vi "Dlg-Add-Exchanges.vi"(8 "error in (no error)":errorcluster, 11 "Exchanges in":refnum<class "Exchanges.lvclass">) -> (0 "error out":errorcluster, 2 "Canceled":bool, 3 "Exchanges out":refnum<class "Exchanges.lvclass">)   [LabVIEW 2012]
uses:
  Exchange/Exchange.lvclass
  Exchange/Exchange Type Enum.ctl
  controls/Currencies.ctl
  Exchange/Exchange Parameters.ctl
  Exchanges.lvclass
  Stocks Manager/Stock Manager Action.ctl
panel:
  in  "Label":string
  in  "ISIN":string
  in  "Taxe":dbl
  in  "Quantité":dbl
  in  "Type":T1
  in  "Currency":T2
  in  "Prix":dbl
  in  "Add":bool
  in  "Date":timestamp format="%<%X\n%x>T"
  in  "Commentaires":string
  in  "Cancel Button":bool
  in  "Help":bool
  # "Nouveau Portefeuille"
  # "Ajouter une Transaction"
  # "Transaction"
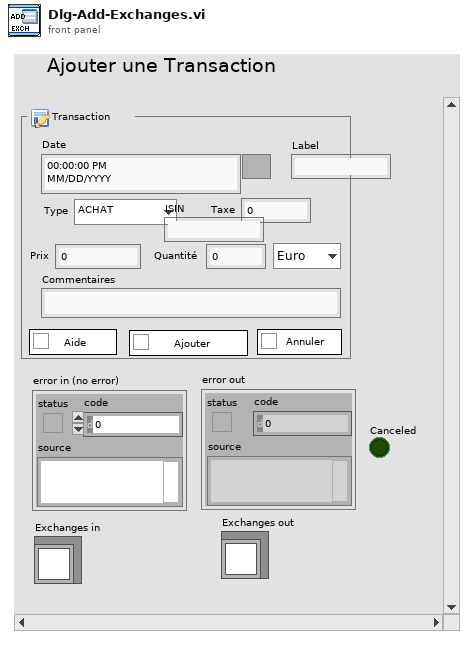
[diagram p1: front panel]
types:
  T1 = typedef "Exchange.lvclass/Exchange Type Enum.ctl" = enum16{"ACHAT", "VENTE"}
  T2 = typedef "Currencies.ctl" = enum16{"Euro", "Dollar", "Yen", "RIM", "CHF"}
  T3 = typedef "Exchange Parameters.ctl" = cluster{"Date":timestamp, "Exchange Type":T1, "ISIN":string, "Label":string, "Price":dbl, "Qty":dbl, "Currency":T2, "Tax":dbl, "Comment":string}
  T4 = typedef "Stock Manager Action.ctl" = enum16{"Get_Stocks", "Load_Stocks", "Find_Stock_From_ISIN", "Find_Stock_From_Label", "Find_Stock_From_Symbol"}
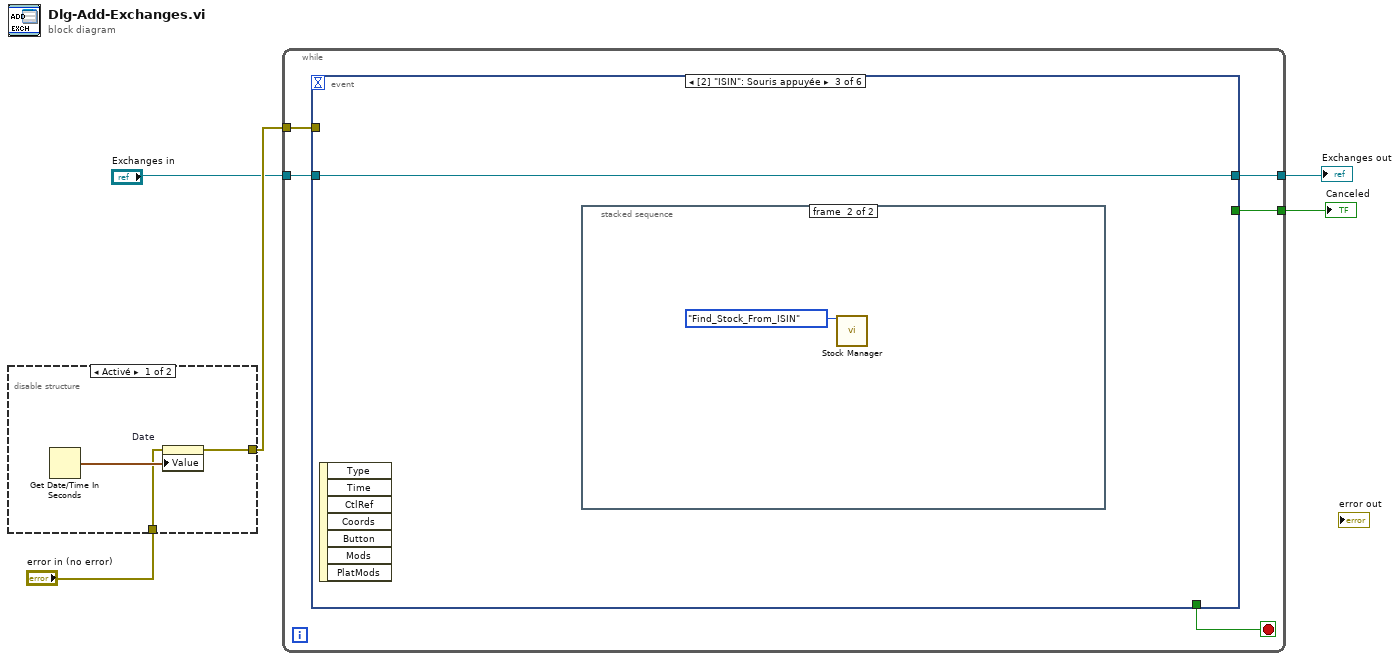
[diagram p0: block diagram]
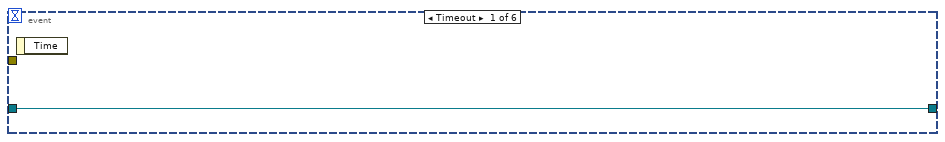
[diagram p2: hidden frame]
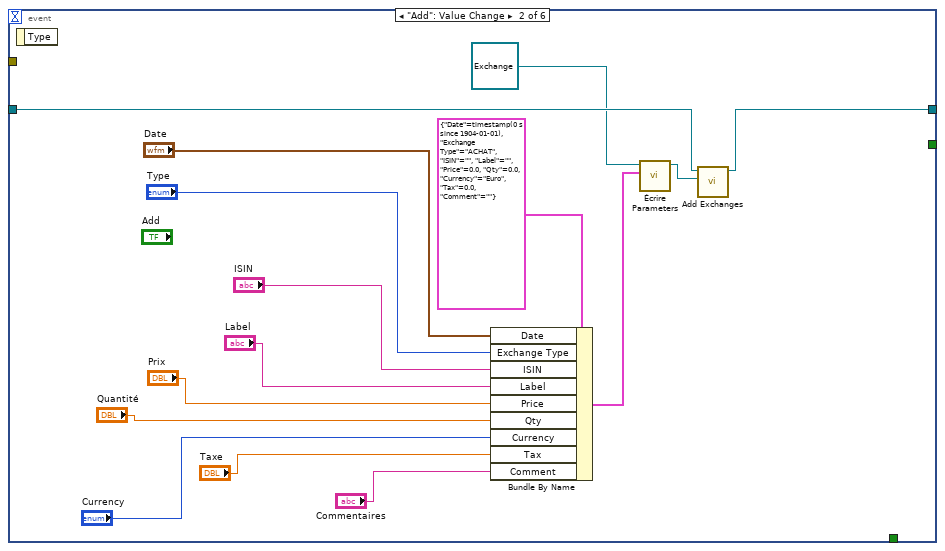
[diagram p3: hidden frame]
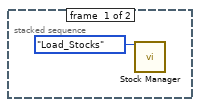
[diagram p4: hidden frame]
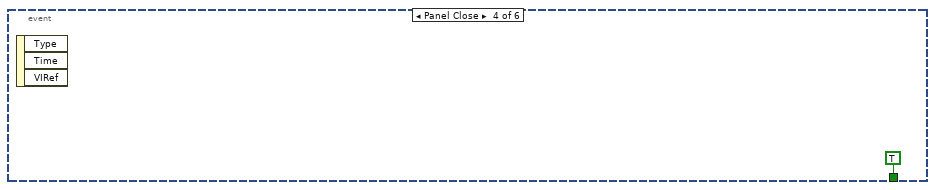
[diagram p5: hidden frame]
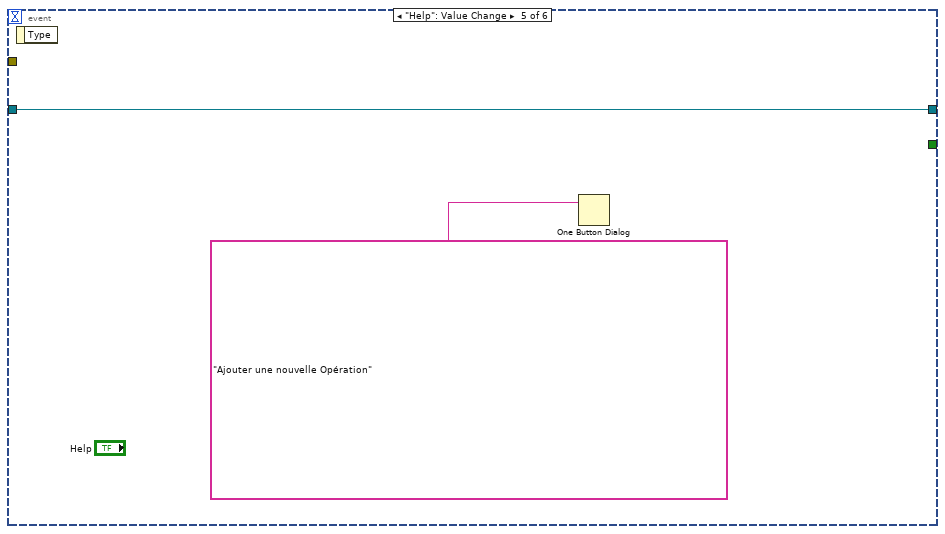
[diagram p6: hidden frame]
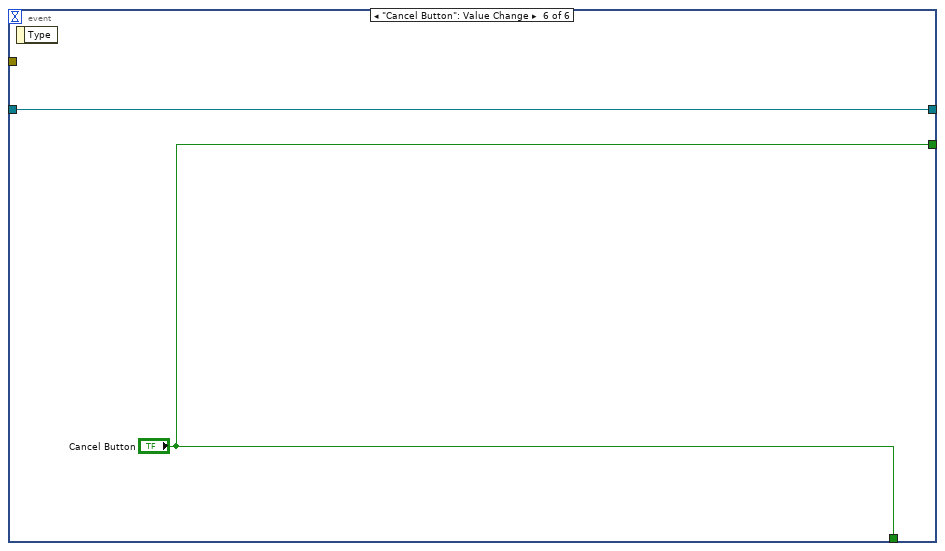
[diagram p7: hidden frame]
diagram:
  n1 = disable-structure shown="Activé" {
    disable-tunnel: [w7 _] -> w5
    disable-tunnel: "error in (no error)" -> [w6 _]
    frame Enabled {
      n2 = Get Date/Time In Seconds() -> (seconds since 1Jan1904=w8:timestamp)
      n3 = property on="Date" class="TempsAbs (strict)"(error in=w6, "Value"=w8) -> (error out=w7:errorcluster)  [unwired: 1 in, 1 out]
    }
    frame Disabled {
    }
  }
  n4 = while {
    tunnel: w5 -> [w13]
    tunnel: [w12] -> w3
    tunnel: "Exchanges in" -> [w11]
    tunnel: [w10] -> w1
    stop <- w9 stop-if-true
    n5 = event shown="[2] \"ISIN\": Souris appuyée" {
      selector: _ -> [_ _ _ _ _ _]
      dyn-events: _ -> [_ _ _ _ _ _]
      timeout: _ -> [_ _ _ _ _ _]
      tunnel: w13 -> [_ _ _ _ _ _]
      tunnel: [_ _ _ _ _ "Cancel Button"] -> w12
      tunnel: w11 -> [w14 w28 w30 _ w34 w37]
      tunnel: [w14 w27 w30 _ w34 w37] -> w10
      tunnel: [_ _ _ TRUE ("Cancel Button") _ "Cancel Button"] -> w9
      event Timeout {
        n6 = event-data() -> ()  [unwired: 1 in, 1 out]
      }
      event "Add": Value Change {
        n7 = event-data() -> ()  [unwired: 1 in, 1 out]
        n8 = Bundle By Name(cluster=T3 {"Date"=timestamp(0 s since 1904-01-01), "Exchange Type"=enum."ACHAT", "ISIN"="", "Label"="", "Price"=0.0, "Qty"=0.0, "Currency"=enum."Euro", "Tax"=0.0, "Comment"=""} ("Parameters"), "Date"="Date", "Exchange Type"="Type", "ISIN"="ISIN", "Label"="Label", "Price"="Prix", "Qty"="Quantité", "Currency"="Currency", "Tax"="Taxe", "Comment"="Commentaires") -> (w23:T3)
        n9 = call "Écrire Parameters.vi"("Parameters"=w23, "Exchange en entrée"=refnum<class "Exchange.lvclass"> refnum ("Exchange.lvclass")) -> ("Exchange en sortie"=w24:refnum<class "Exchange.lvclass">)  [unwired: 9 in]
        n10 = call "Add Exchanges.vi"("Exchange Added"=w24, "Exchanges en entrée"=w28) -> ("Exchanges en sortie"=w27:refnum<class "Exchanges.lvclass">)  [unwired: 7 in, 2 out]
      }
      event "ISIN": Mouse Down {
        n11 = event-data() -> ()  [unwired: 1 in, 7 out]
        n12 = stacked-sequence {
          frame #0 {
            n13 = call "Stock Manager.vi"("Stock Manager Action"=Stock_Manager_Action."Load_Stocks") -> ()  [unwired: 11 in, 4 out]
          }
          frame #1 {
            n14 = call "Stock Manager.vi"("Stock Manager Action"=Stock_Manager_Action."Find_Stock_From_ISIN") -> ()  [unwired: 11 in, 4 out]
          }
        }
      }
      event Panel Close {
        n15 = event-data() -> ()  [unwired: 1 in, 3 out]
      }
      event "Help": Value Change {
        n16 = event-data() -> ()  [unwired: 1 in, 1 out]
        n17 = One Button Dialog(message="Ajouter une nouvelle Opération") -> ()  [unwired: 1 in, 1 out]
      }
      event "Cancel Button": Value Change {
        n18 = event-data() -> ()  [unwired: 1 in, 1 out]
      }
    }
  }
  "Canceled" <- w3
  "Exchanges out" <- w1
